vi "Fetch&Process_Measurements_V3.vi"(8 "error in (no error)":errorcluster, 9 "Initial Time":timestamp, 10 "DCPowerInformation_byChannel":T1(array[cluster]), 11 "DCPowerDataQueueControl_V2 in":T2) -> (0 "error out":errorcluster, 1 "Current Waveform":waveform(dbl)[](array[waveform]), 2 "Voltage Waveform":waveform(dbl)[](array[waveform]), 3 "DCPowerDataQueueControl_V2 out":T2)   [LabVIEW 2019]
uses:
  Controls/QueueDataControl_V2.ctl
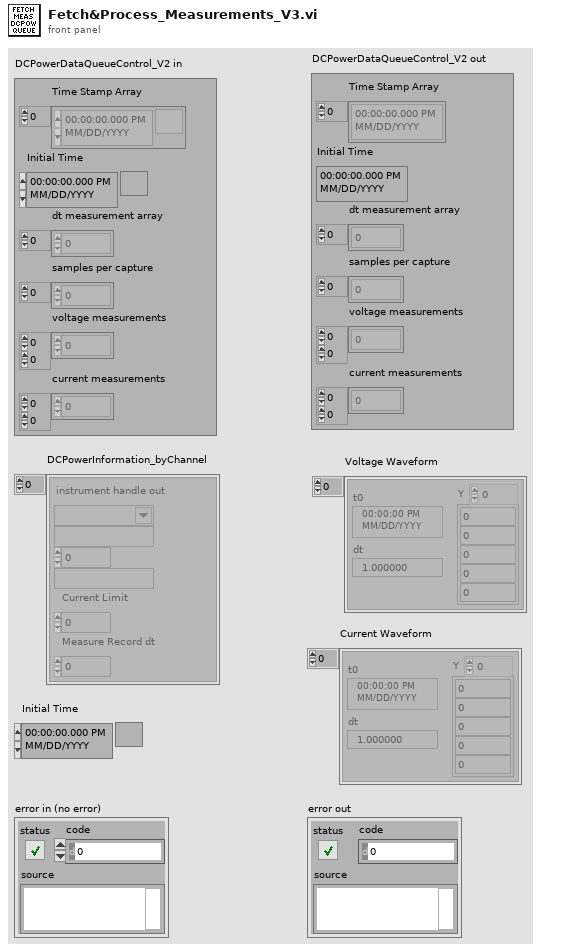
[diagram p1: front panel]
types:
  T1 = cluster{"instrument handle out":refnum<k15>, string, dbl, string, "Current Limit":dbl, "Measure Record dt":dbl}[]
  T2 = typedef "QueueDataControl_V2.ctl" = cluster{"Time Stamp Array":timestamp[], "Initial Time":timestamp, "dt measurement array":dbl[], "samples per capture":i32[], "voltage measurements":dbl[][], "current measurements":dbl[][]}
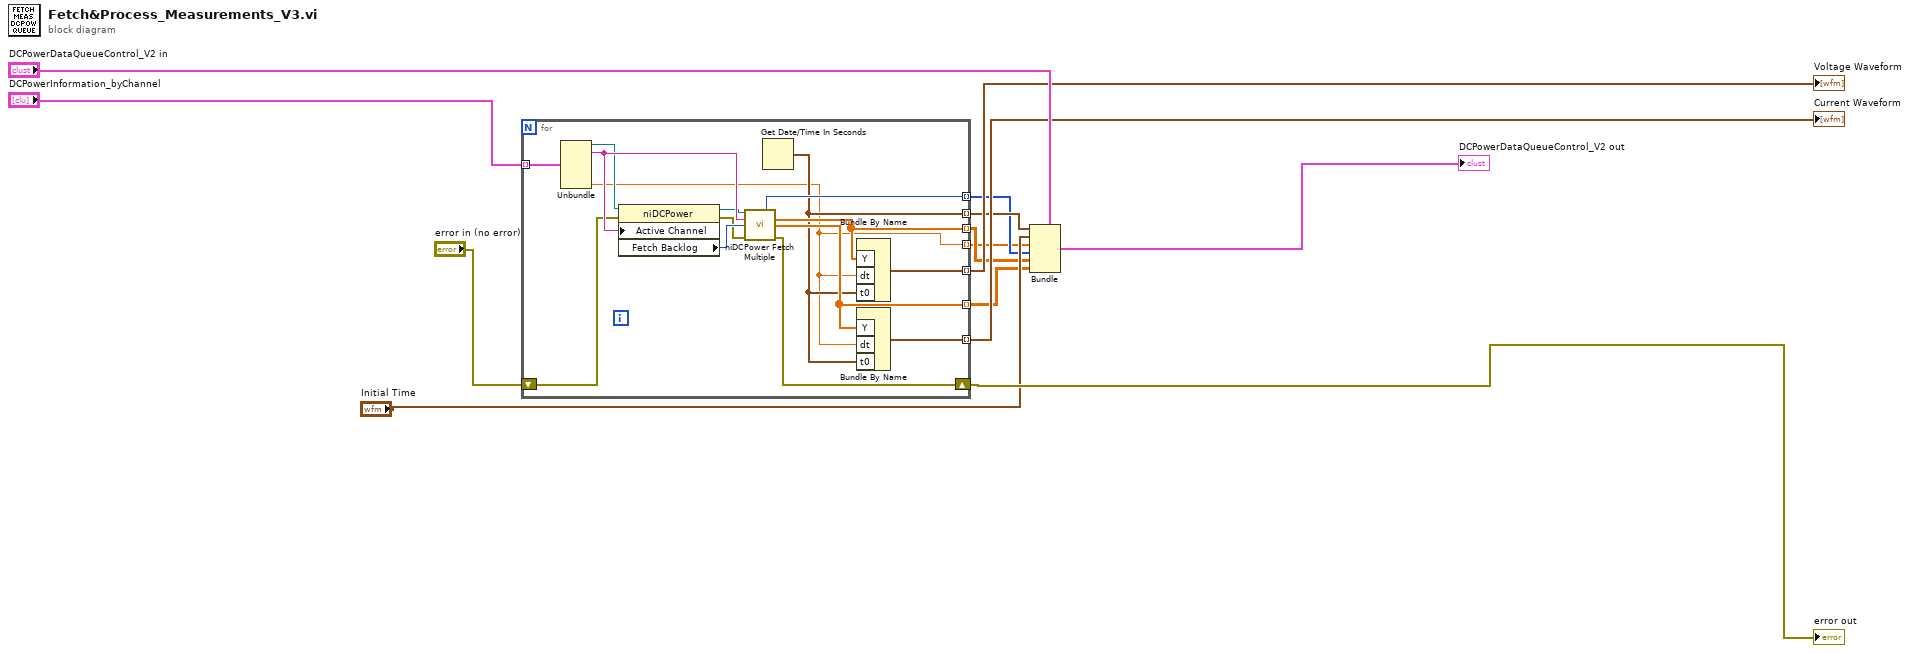
[diagram p0: block diagram]
diagram:
  n1 = for {
    tunnel: "DCPowerInformation_byChannel" -> [w28] mode=indexing
    tunnel: [w21] -> w7 mode=indexing
    tunnel: [w20] -> w8 mode=indexing
    tunnel: [w19] -> w3 mode=indexing
    tunnel: [w18] -> w5 mode=indexing
    tunnel: [w17] -> w4 mode=indexing
    tunnel: [w16] -> w6 mode=indexing
    tunnel: [w15] -> w2 mode=indexing
    shift-right: [w14] -> w13
    shift-left: "error in (no error)" -> [w25]
    n2 = Unbundle(w28) -> ("instrument handle out"=w24:refnum<k15>, w27:string, "Measure Record dt"=w15:dbl)  [unwired: 3 out]
    n3 = property class="niDCPower"(reference=w24, error in=w25, "Active Channel"=w27) -> (reference out=w23:refnum<k15>, error out=w22:errorcluster, "Fetch Backlog"=w26:i32)
    n4 = call <instrlib>:"niDCPower Fetch Multiple.vi"("instrument handle"=w23, "channel name"=w27, "count (1)"=w26, "error in (no error)"=w22) -> ("actual count"=w19:i32, "voltage measurements"=w17:dbl[], "current measurements"=w18:dbl[], "error out"=w14:errorcluster)  [unwired: 6 in, 2 out]
    n5 = Get Date/Time In Seconds() -> (seconds since 1Jan1904=w16:timestamp)
    n6 = Bundle By Name("Y"=w17, "dt"=w15, "t0"=w16) -> (w21:waveform(dbl))  [unwired: 1 out]
    n7 = Bundle By Name("Y"=w18, "dt"=w15, "t0"=w16) -> (w20:waveform(dbl))  [unwired: 1 out]
  }
  "error out" <- w13
  "Current Waveform" <- w8
  "Voltage Waveform" <- w7
  n8 = Bundle(cluster="DCPowerDataQueueControl_V2 in", "Time Stamp Array"=w6, "Initial Time"="Initial Time", "dt measurement array"=w2, "samples per capture"=w3, "voltage measurements"=w4, "current measurements"=w5) -> (→"DCPowerDataQueueControl_V2 out":T2)
